vi "Exit case.vi"(8 "error in":errorcluster, 9 "UI queue":refnum<queue>, 11 "Acq. queue":refnum<queue>) -> (0 "error out":errorcluster, 1 "Exit String":string="Exit", 3 "Acq. queue (out)":refnum<queue>)   [LabVIEW 2017]
uses:
  Queue/Message Queue/Typedefs/Message Cluster.ctl
  Typedefs/Read Write Enum.ctl
  Global Variables/gl_UI Ctrl Refs.vi
  Global Variables/General Globals.vi
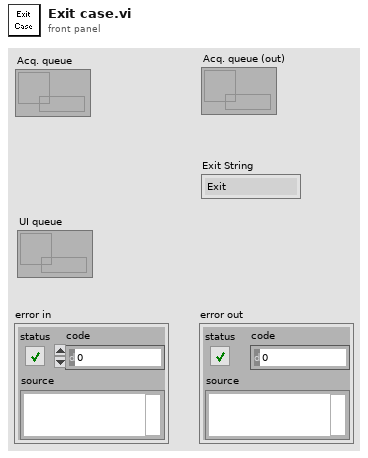
[diagram p1: front panel]
types:
  T1 = typedef "Read Write Enum.ctl" = enum16{"Read", "Write"}
  T2 = typedef "UI ctrl refs cluster.ctl" = cluster{"Top level VI path":path, "Top level VI ref":refnum<vi>, "User menu ref":refnum<k9>, "Sub Panel control":refnum<vi>, "Imaging Param Tab":refnum<vi>, "Occurrence-Start drivers":refnum<k4>, "Occurrence-Speed logging initialised":refnum<k4>, "Occurrence-XYZ stage initialised":refnum<k4>, "Exit button":refnum<vi>, "Status ind":refnum<vi>, "Set as origin":refnum<vi>, "Speed Logging":refnum<vi>, "Time Lapse":refnum<vi>, "Live Imaging":refnum<vi>, "AOL Z Stack":refnum<vi>, "Motor Z Stack":refnum<vi>, "Funct Acq button":refnum<vi>, "Hard Shutter":refnum<vi>, "Virtual Shutter":refnum<vi>, "Laser Power":refnum<vi>, "AOL Mode":refnum<vi>, "Frame Size":refnum<vi>, "Field of View":refnum<vi>, "Dwell Time":refnum<vi>, "Zoom":refnum<vi>, "AOL Z":refnum<vi>, "Objective":refnum<vi>, "Axis":refnum<vi>, "Paths & Names":refnum<vi>, "Experiment folder path (ind.)":refnum<vi>, "Last State (Ind.)":refnum<vi>, "Laser wavelength ind (nm)":refnum<vi>, "Averages":refnum<vi>, "Angle (degrees)":refnum<vi>, "X centre":refnum<vi>, "Y centre":refnum<vi>, "Plane Mode":refnum<vi>, "# Planes":refnum<vi>, "Z Start":refnum<vi>, "Z Stop":refnum<vi>, "Z Step":refnum<vi>, "PMT 1":refnum<vi>, "PMT 2":refnum<vi>, "Stage XYZ Position":refnum<vi>, "Pockels@Z Start":refnum<vi>, "Pockels@Z Stop":refnum<vi>, "Obtain Z Start":refnum<vi>, "Obtain Z Stop":refnum<vi>, "Live stim.trig.period":refnum<vi>, "Live stim.trig.enable":refnum<vi>, "Movement Correction":refnum<vi>, "Load Reference Image":refnum<vi>, "XY Stage Move":refnum<vi>, "MovCor Cluster":refnum<vi>, "RefDAQParam":refnum<vi>, "Funct. Acq. Pockels Modulation":refnum<vi>, "Background MovCor":refnum<vi>, "Ref Laser Power":refnum<vi>, "Enable Video Recording":refnum<vi>, "Video Record-Live Imaging":refnum<vi>, "Video Record-Funct acq":refnum<vi>, "Reference Source":refnum<vi>, "AOL Z-stack Chirps Ready (ind)":refnum<vi>, "Target time between mov.cor. ref triggers (ms)":refnum<vi>, "Funct. Acq. Ref frame save":refnum<vi>, "Tracking button":refnum<vi>, "Show ref plots window":refnum<vi>, "Center freq ind (nm)":refnum<vi>, "Pickup mode (ind)":refnum<vi>, "Logging queue (ind)":refnum<vi>, "Back aperture power (ind.)":refnum<vi>, "Power after objective (ind.)":refnum<vi>, "Switch user":refnum<vi>}
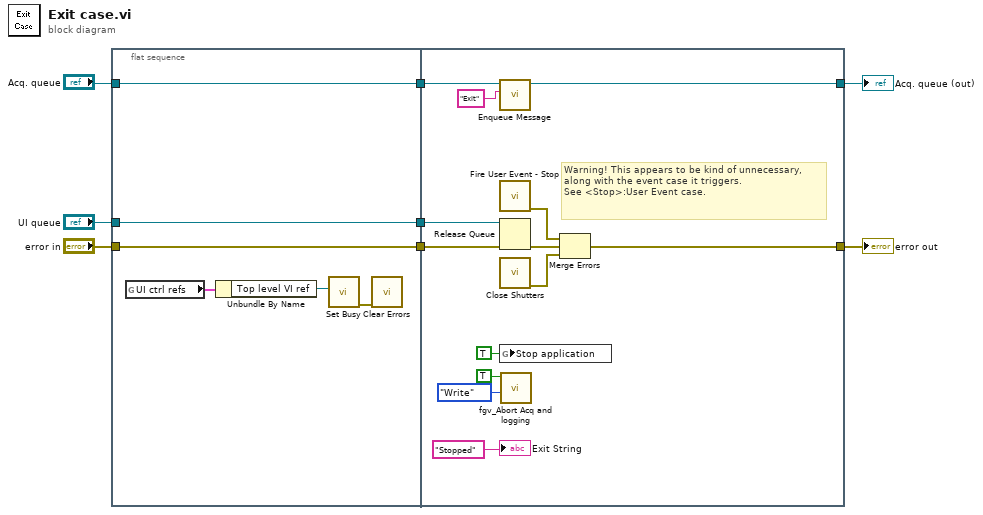
[diagram p0: block diagram]
diagram:
  n1 = flat-sequence {
    tunnel: "UI queue" -> [w12]
    tunnel: "Acq. queue" -> [w13]
    tunnel: "error in" -> [w14]
    tunnel: [w14] -> w3
    tunnel: [w13] -> w2
    tunnel: [w12] -> w1
    tunnel: [w24] -> w8
    tunnel: [w18] -> w5
    tunnel: w3 -> [w20]
    tunnel: w2 -> [w19]
    tunnel: w1 -> [w17]
    frame #0 {
      n2 = global read "gl_UI Ctrl Refs.vi" "UI ctrl refs"() -> (w9:T2)
      n3 = Unbundle By Name(w9) -> ("Top level VI ref"=w10:refnum<vi>)
      n4 = call <vilib>:"Set Busy.vi"("VI reference (current VI)"=w10) -> ("error out"=w11:errorcluster)  [unwired: 9 in, 1 out]
      n5 = call <vilib>:"Clear Errors.vi"("error in (no error)"=w11) -> ()  [unwired: 5 in, 2 out]
    }
    frame #1 {
      # "Warning! This appears to be kind of unnecessary, along with the event case it triggers.\nSee <Stop>:User Event case."
      n6 = call "Enqueue Message.vi"("Message"="Exit", "Queue"=w19) -> ("Queue out"=w18:refnum<queue>)  [unwired: 8 in, 1 out]
      n7 = call "Fire User Event - Stop.vi"() -> ("Error Out"=w21:errorcluster)  [unwired: 11 in]
      n8 = Release Queue(queue=w17, error in (no error)=w20) -> (error out=w23:errorcluster)  [unwired: 1 in, 2 out]
      n9 = call "Close Shutters.vi"() -> ("error out (no error)"=w25:errorcluster)  [unwired: 11 in]
      n10 = global write "General Globals.vi" "Stop application"(TRUE ("Stop application")) -> ()
      n11 = call "fgv_Abort Acq and logging.vi"("Function"=Read_Write_Enum."Write", "Live Imaging?"=TRUE) -> ()  [unwired: 8 in, 2 out]
      n12 = Merge Errors(w21, w23, w25) -> (w24:errorcluster)
      "Exit String" <- "Stopped" ("Exit String")
    }
  }
  "error out" <- w8
  "Acq. queue (out)" <- w5
